vi "Read Module Tree.vi"(8 "error in (no error)":errorcluster, 11 "Startup.ini":path) -> (0 "error out":errorcluster, 2 "Items":T1(array[cluster]), 3 "Startup.ini out":path)   [LabVIEW 2022 SP3, in "Core.lvlib" / "Config.lvlib"]
uses:
  Config.lvlib
  <vilib>/Utility/config.llb/NI_LVConfig.lvlib
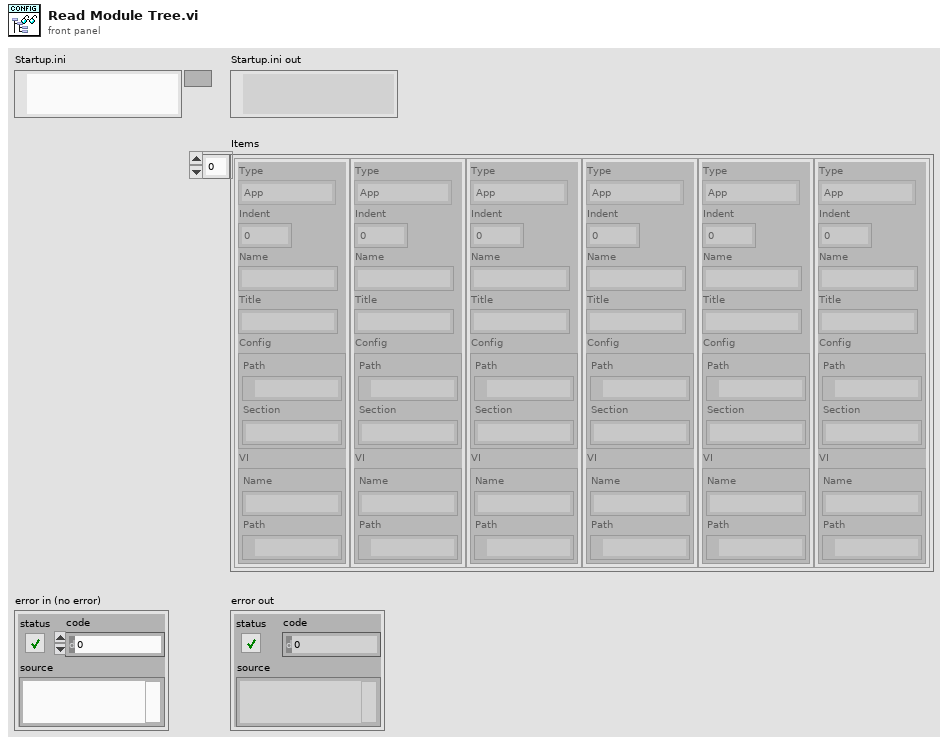
[diagram p1: front panel]
types:
  T1 = cluster{"Type":enum8{"App", "Module", "ModuleGroup"}, "Indent":i32, "Name":string, "Title":string, "Config":cluster{"Path":path, "Section":string}, "VI":cluster{"Name":string, "Path":path}}[]
  T2 = typedef "NI_LVConfig.lvlib/Config Data RefNum.ctl" = refnum<k1>
  T3 = cluster{"Type":enum8{"App", "Module", "ModuleGroup"}, "Indent":i32, "Name":string, "Title":string, "Config":cluster{"Path":path, "Section":string}, "VI":cluster{"Name":string, "Path":path}}
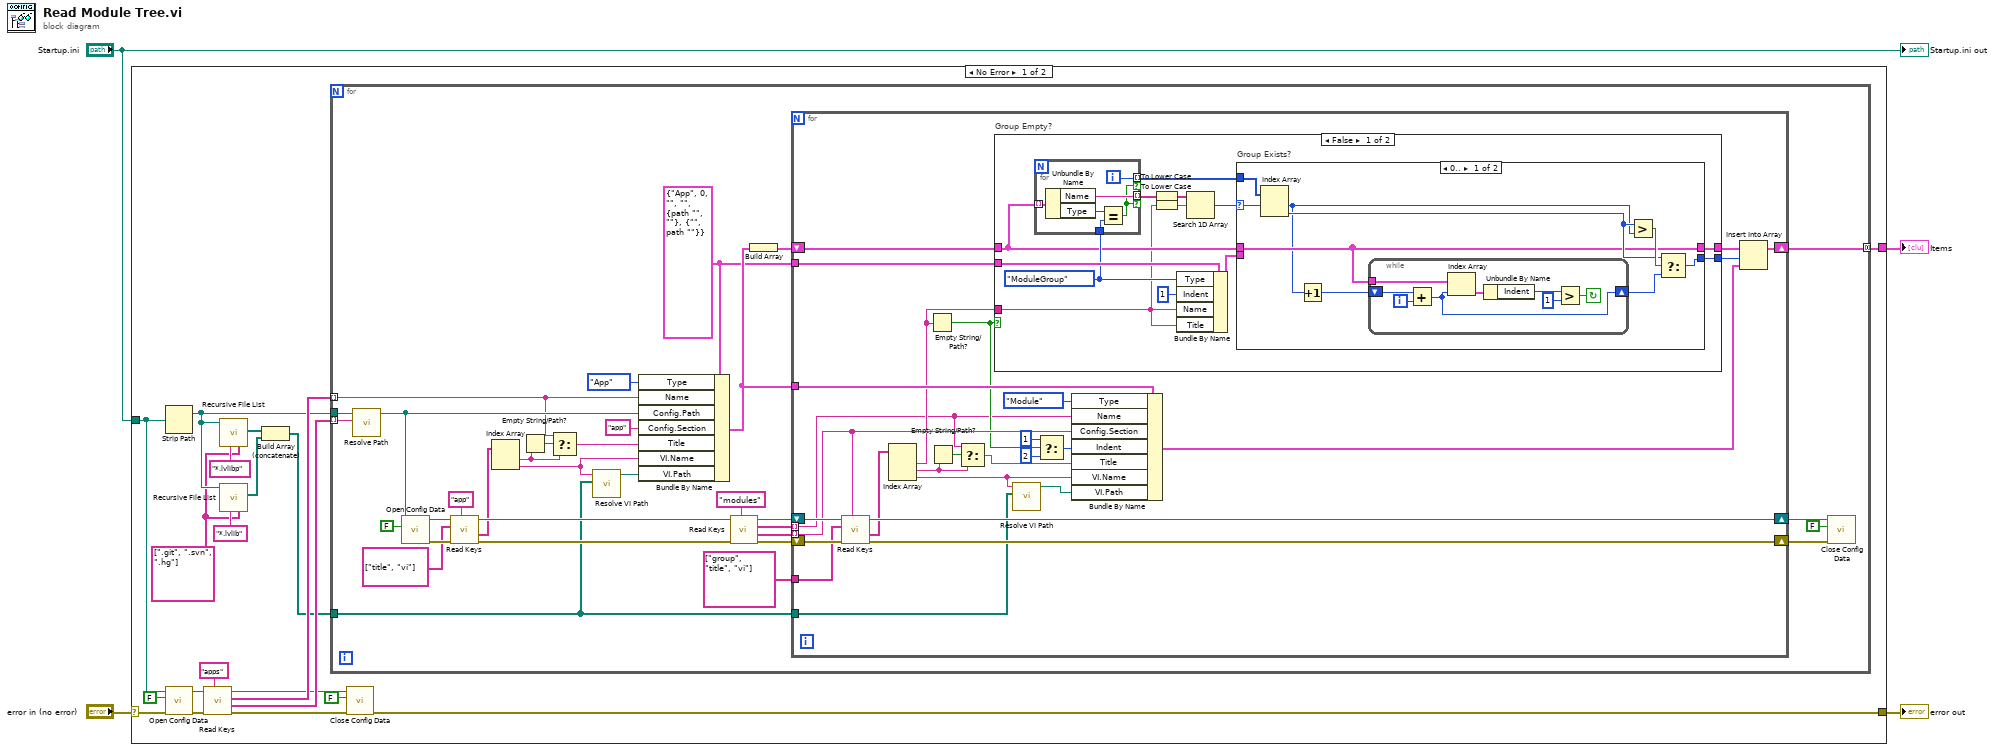
[diagram p0: block diagram]
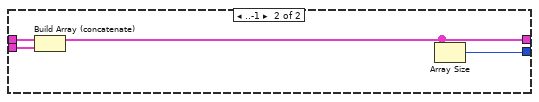
[diagram p2: hidden frame]
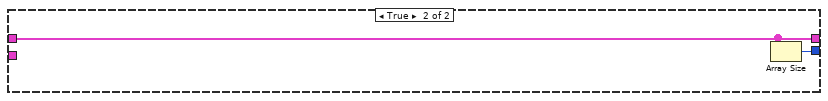
[diagram p3: hidden frame]
diagram:
  n1 = case shown="No Error" "error in (no error)" {
    selector: "error in (no error)" -> [w17 w127]
    tunnel: "Startup.ini" -> [w18 _]
    tunnel: [w13 w127] -> w3
    tunnel: [w12 _] -> w2
    frame No Error {
      w5 = string[] [".git", ".svn", ".hg"] ("Folders to Exclude")
      n2 = Strip Path(path=w18) -> (stripped path=w11:path)  [unwired: 1 out]
      n3 = call <vilib>:"Open Config Data.vi"("error in (no error)"=w17, "create file if necessary (T)"=FALSE, "configuration file path"=w18) -> ("error out"=w16:errorcluster, "refnum"=w15:T2)  [unwired: 6 in, 1 out]
      n4 = call "Read Keys.vi"("Section"="apps", "error in (no error)"=w16, "Config Refnum in"=w15) -> ("error out"=w21:errorcluster, "Values"=w23:string[], "Key Names"=w22:string[], "Config Refnum out"=w20:T2)  [unwired: 4 in, 1 out]
      n5 = call <vilib>:"Recursive File List.vi"("Folders to Exclude"=w5, "pattern"="*.lvlibp", "Folder Path"=w11) -> ("All Files in Dir"=w10:path[])  [unwired: 4 in, 4 out]
      n6 = call <vilib>:"Recursive File List.vi"("Folders to Exclude"=w5, "pattern"="*.lvlib", "Folder Path"=w11) -> ("All Files in Dir"=w9:path[])  [unwired: 4 in, 4 out]
      n7 = Build Array (concatenate)(w10, w9) -> (w6:path[])
      n8 = for {
        tunnel: w11 -> [w55]
        tunnel: w23 -> [w54] mode=indexing
        tunnel: w22 -> [w25] mode=indexing
        tunnel: [w31] -> w12 mode=concatenating
        tunnel: w6 -> [w30]
        w29 = T3 {"Type"=enum."App", "Indent"=0, "Name"="", "Title"="", "Config"={"Path"=path "", "Section"=""}, "VI"={"Name"="", "Path"=path ""}} ("Item")
        n9 = call "Resolve Path.vi"("Path"=w54, "Base Dir"=w55) -> ("Resolved Path"=w37:path)  [unwired: 9 in]
        n10 = call <vilib>:"Open Config Data.vi"("create file if necessary (T)"=FALSE, "configuration file path"=w37) -> ("error out"=w53:errorcluster, "refnum"=w52:T2)  [unwired: 7 in, 1 out]
        n11 = call "Read Keys.vi"("Section"="app" ("section"), "error in (no error)"=w53, "Key Names ([]=All Keys)"=string[] ["title", "vi"], "Config Refnum in"=w52) -> ("error out"=w49:errorcluster, "Values"=w46:string[], "Config Refnum out"=w48:T2)  [unwired: 3 in, 2 out]
        n12 = Index Array(array=w46) -> (element #1=w28:string, element #2=w33:string)  [unwired: 2 in]
        n13 = Empty String/Path?(string/path=w28) -> (empty?=w27:bool)
        n14 = Select(t=w25, s=w27, f=w28) -> (s? t:f=w26:string)
        n15 = call "Resolve VI Path.vi"("Library Paths (.lvlibp, .lvlib)"=w30, "Qualified Name (lvlibp|lvlib[:vi])"=w33) -> ("VI Path"=w32:path)  [unwired: 8 in, 1 out]
        n16 = Bundle By Name(cluster=w29, "Type"=enum8{"App", "Module", "ModuleGroup"}."App", "Name"=w25, "Config.Path"=w37, "Config.Section"="app", "Title"=w26, "VI.Name"=w33, "VI.Path"=w32) -> (w34:T3)
        n17 = call "Read Keys.vi"("Section"="modules", "error in (no error)"=w49, "Config Refnum in"=w48) -> ("error out"=w45:errorcluster, "Values"=w40:string[], "Key Names"=w41:string[], "Config Refnum out"=w44:T2)  [unwired: 4 in, 1 out]
        n18 = Build Array(w34) -> (w35:T1)
        n19 = for {
          shift-right: [w82] -> w43
          shift-left: w45 -> [w84]
          shift-right: [w81] -> w42
          shift-left: w44 -> [w83]
          tunnel: w41 -> [w59] mode=indexing
          tunnel: w40 -> [w71] mode=indexing
          tunnel: string[] ["group", "title", "vi"] ("Key Names ([]=All Keys)") -> [w80]
          shift-right: [w77] -> w31
          shift-left: w35 -> [w64]
          tunnel: w34 -> [w79]
          tunnel: w30 -> [w68]
          tunnel: w29 -> [w67]
          n20 = call "Read Keys.vi"("Section"=w71, "error in (no error)"=w84, "Key Names ([]=All Keys)"=w80, "Config Refnum in"=w83) -> ("error out"=w82:errorcluster, "Values"=w75:string[], "Config Refnum out"=w81:T2)  [unwired: 3 in, 2 out]
          n21 = Index Array(array=w75) -> (element #1=w66:string, element #2=w60:string, element #3=w70:string)  [unwired: 3 in]
          n22 = Empty String/Path?(string/path=w66) -> (empty?=w63:bool)
          n23 = Empty String/Path?(string/path=w60) -> (empty?=w61:bool)
          n24 = Select(t=w59, s=w61, f=w60) -> (s? t:f=w58:string)
          n25 = case "Group Empty?" shown="False" w63 {
            tunnel: w67 -> [w97 _]
            tunnel: w66 -> [w85 _]
            tunnel: [w91 w125] -> w65
            tunnel: w64 -> [w90 w125]
            tunnel: [w87 w126] -> w62
            frame False {
              w95 = enum8{"App", "Module", "ModuleGroup"}."ModuleGroup" ("Type")
              n26 = for {
                tunnel: w90 -> [w124] mode=indexing
                tunnel: [w123] -> w86 mode=indexing if=w120
                tunnel: [w122] -> w94 mode=indexing if=w120
                tunnel: w95 -> [w121]
                i -> [w123]
                n27 = Unbundle By Name(w124) -> ("Name"=w122:string, "Type"=w119:enum8{"App", "Module", "ModuleGroup"})
                n28 = Equal?(x=w119, y=w121) -> (x = y?=w120:bool)
              }
              n29 = To Lower Case(string=w94) -> (all lower case string=w93:string[])
              n30 = To Lower Case(string=w85) -> (all lower case string=w92:string)
              n31 = Bundle By Name(cluster=w97, "Type"=w95, "Indent"=1, "Name"=w85, "Title"=w85) -> (w89:T3)
              n32 = Search 1D Array(1D array=w93, element=w92) -> (index of element=w88:i32)  [unwired: 1 in]
              n33 = case "Group Exists?" shown="0.." w88 {
                selector: w88 -> [w105 _]
                tunnel: [w101 w116] -> w91
                tunnel: w90 -> [w101 w118]
                tunnel: w89 -> [_ w117]
                tunnel: [w102 w115] -> w87
                tunnel: w86 -> [w106 _]
                frame 0.. {
                  n34 = Index Array(array=w106, index #1=w105) -> (element #1=w100:i32, element #2=w103:i32)  [unwired: 1 in]
                  n35 = Increment(x=w100) -> (x+1=w99:i32)
                  n36 = while {
                    tunnel: w101 -> [w114]
                    shift-right: [w108] -> w98
                    shift-left: w99 -> [w113]
                    i -> [w109]
                    stop <- w107 continue-if-true
                    n37 = Add(x=w113, y=w109) -> (x+y=w108:i32)
                    n38 = Index Array(array=w114, index=w108) -> (element=w112:T3)
                    n39 = Unbundle By Name(w112) -> ("Indent"=w111:i32)
                    n40 = Greater?(x=w111, y=1) -> (0:w107:bool)
                  }
                  n41 = Greater?(x=w103, y=w100) -> (0:w104:bool)
                  n42 = Select(t=w103, s=w104, f=w98) -> (s? t:f=w102:i32)
                }
                frame ..-1 {
                  n43 = Build Array (concatenate)(w118, w117) -> (w116:T1)
                  n44 = Array Size(array=w116) -> (size(s)=w115:i32)
                }
              }
            }
            frame True {
              n45 = Array Size(array=w125) -> (size(s)=w126:i32)
            }
          }
          n46 = call "Resolve VI Path.vi"("Library Paths (.lvlibp, .lvlib)"=w68, "Qualified Name (lvlibp|lvlib[:vi])"=w70) -> ("VI Path"=w69:path)  [unwired: 8 in, 1 out]
          n47 = Select(t=1, s=w63, f=2) -> (s? t:f=w72:i32)
          n48 = Bundle By Name(cluster=w79, "Type"=enum8{"App", "Module", "ModuleGroup"}."Module", "Name"=w59, "Config.Section"=w71, "Indent"=w72, "Title"=w58, "VI.Name"=w70, "VI.Path"=w69) -> (w76:T3)
          n49 = Insert Into Array(array=w65, index=w62, new element=w76) -> (w77:T1)
        }
        n50 = call <vilib>:"Close Config Data.vi"("error in (no error)"=w43, "write file if changed (T)"=FALSE, "refnum"=w42) -> ()  [unwired: 7 in, 2 out]
      }
      n51 = call <vilib>:"Close Config Data.vi"("error in (no error)"=w21, "write file if changed (T)"=FALSE, "refnum"=w20) -> ("error out"=w13:errorcluster)  [unwired: 7 in, 1 out]
    }
    frame Error {
    }
  }
  "error out" <- w3
  "Items" <- w2
  "Startup.ini out" <- "Startup.ini"
